vi "Create Custom Device Config Storage.vi"(8 "error in":errorcluster, 11 "Document Element":refnum<k20>) -> (0 "error out":errorcluster, 2 "Custom Device Config out":refnum<class "Custom Device Config.lvclass">, 3 "Document Element":refnum<k20>)   [LabVIEW 2024, in "Parser.lvlib" / "Custom Device Config.lvclass"]
uses:
  Custom Device Config.lvclass
  C:/dev/CD/niveristand-fpga-addon-custom-device/Source/Addon/Parser/Item/Item.lvclass
  Item/Controls/Item Type.ctl
  Property/Property.lvclass
  Custom Device Config.lvclass/Custom Device Config.ctl
  Item/Item.lvclass/Item.ctl
  Write XSDVersion.vi
  Write Version.vi
  Item/Write Child Items.vi
  Item/Write Properties.vi
  Write Name.vi
  <vilib>/xml/Close Reference(Node).vi
  <resource>/objmgr/DOMUserDefRef.rc
  <vilib>/xml/NI_XML.lvlib
  Item/Item.lvclass
  Parser.lvlib
  Channel/Channel.lvclass
  Section/Section.lvclass
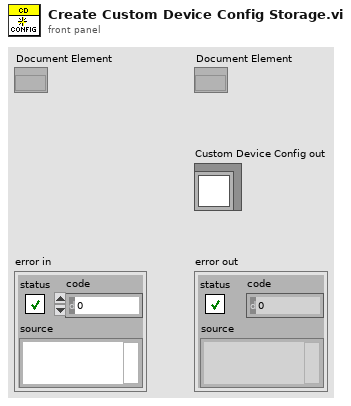
[diagram p1: front panel]
types:
  T1 = cluster{"Major":u32, " Minor":u32, " Fix":u32, "Build":u32}
  T2 = typedef "Parser.lvlib/Item.lvclass/Item Type.ctl" = enum16{"Channel", "Section"}
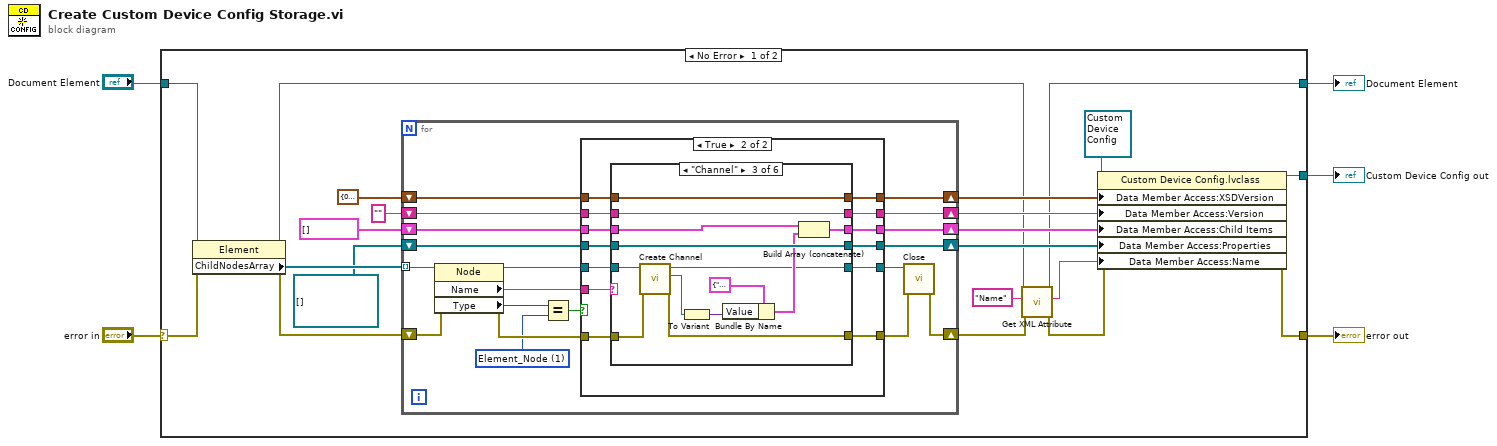
[diagram p0: block diagram]
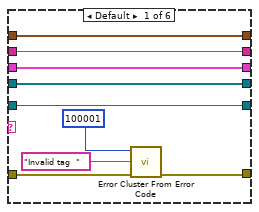
[diagram p3: hidden frame]
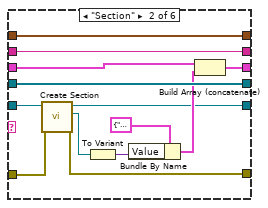
[diagram p4: hidden frame]
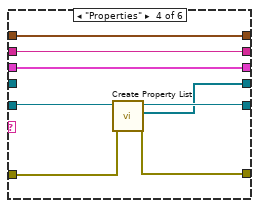
[diagram p5: hidden frame]
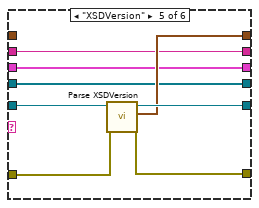
[diagram p6: hidden frame]
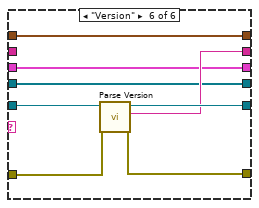
[diagram p7: hidden frame]
diagram:
  n1 = case shown="No Error" "error in" {
    selector: "error in" -> [w25 w125]
    tunnel: [w20 _] -> w3
    tunnel: [w26 w125] -> w5
    tunnel: "Document Element" -> [w19 w124]
    tunnel: [w7 w124] -> w1
    frame No Error {
      n2 = property class="Element"(reference=w19, error in=w25) -> (reference out=w8:refnum<k20>, error out=w24:errorcluster, "ChildNodesArray"=w12:refnum<k20>[])
      n3 = for {
        tunnel: w12 -> [w41] mode=indexing
        shift-right: [w44] -> w23
        shift-left: w24 -> [w45]
        shift-right: [w36] -> w18
        shift-left: T1 {"Major"=0, " Minor"=0, " Fix"=0, "Build"=0} ("XSDVersion") -> [w32]
        shift-right: [w35] -> w17
        shift-left: "" ("Version") -> [w33]
        shift-right: [w27] -> w16
        shift-left: cluster{"Item Type":T2, "Value":variant}[] [] ("Child Items") -> [w34]
        shift-right: [w29] -> w10
        shift-left: refnum<class "Property.lvclass">[] [] ("Properties") -> [w28]
        w38 = 1 items=["Element_Node"=1, "Attribute_Node"=2, "Text_Node"=3, "CDATASection_Node"=4, "EntityReference_Node"=5, "Entity_Node"=6, "ProcessingInstruction_Node"=7, "Comment_Node"=8, "Document_Node"=9, "DocumentType_Node"=10, "DocumentFragment_Node"=11, "Notation_Node"=12] ("Node Type")
        n4 = property class="Node"(reference=w41, error in=w45) -> (reference out=w39:refnum<k20>, error out=w43:errorcluster, "Name"=w31:string, "Type"=w30:i32)
        n5 = Equal?(x=w30, y=w38) -> (x = y?=w40:bool)
        n6 = case shown="True" w40 {
          tunnel: w31 -> [_ w62]
          tunnel: w39 -> [w50 w61]
          tunnel: [w50 w60] -> w37
          tunnel: w43 -> [w51 w64]
          tunnel: [w51 w63] -> w42
          tunnel: [w49 w59] -> w36
          tunnel: [w48 w58] -> w35
          tunnel: w34 -> [w46 w57]
          tunnel: w33 -> [w48 w56]
          tunnel: w32 -> [w49 w55]
          tunnel: [w47 w54] -> w29
          tunnel: w28 -> [w47 w53]
          tunnel: [w46 w52] -> w27
          frame False {
          }
          frame True {
            n7 = case shown="\"Channel\"" w62 {
              tunnel: w61 -> [w68 w84 w93 w103 w113 w121]
              tunnel: [w68 w74 w87 w102 w112 w120] -> w60
              tunnel: w64 -> [w73 w86 w99 w107 w115 w123]
              tunnel: [w72 w85 w98 w106 w114 w122] -> w63
              tunnel: [w71 w81 w97 w105 w111 w118] -> w59
              tunnel: [w70 w82 w96 w104 w110 w119] -> w58
              tunnel: w57 -> [w65 w83 w95 w100 w108 w116]
              tunnel: w56 -> [w70 w82 w96 w104 w110 _]
              tunnel: w55 -> [w71 w81 w97 w105 _ w118]
              tunnel: [w69 w80 w94 w101 w109 w117] -> w54
              tunnel: w53 -> [w69 w80 w94 _ w109 w117]
              tunnel: [w65 w76 w89 w100 w108 w116] -> w52
              frame Default {
                n8 = call <vilib>:"Error Cluster From Error Code.vi"("error in (no error)"=w73, "error message (\"\")"="Invalid tag  " ("error message (\"\")"), "error code (0)"=100001) -> ("error out"=w72:errorcluster)  [unwired: 6 in]
              }
              frame "Section" {
                n9 = call "Create Section.vi"("error in"=w86, "Node In"=w84) -> ("error out"=w85:errorcluster, "Section out"=w75:refnum<class "Section.lvclass">, "Node out"=w74:refnum<k20>)  [unwired: 7 in]
                n10 = To Variant(anything=w75) -> (Variant=w78:variant)
                n11 = Bundle By Name(cluster=cluster{"Item Type":T2, "Value":variant} {"Item Type"=enum."Section", "Value"=variant} ("Child Items"), "Value"=w78) -> (w77:cluster{"Item Type":T2, "Value":variant})
                n12 = Build Array (concatenate)(w83, w77) -> (w76:cluster{"Item Type":T2, "Value":variant}[])
              }
              frame "Channel" {
                n13 = call "Create Channel.vi"("error in"=w99, "Node In"=w93) -> ("error out"=w98:errorcluster, "Channel out"=w88:refnum<class "Channel.lvclass">, "Node out"=w87:refnum<k20>)  [unwired: 7 in]
                n14 = To Variant(anything=w88) -> (Variant=w91:variant)
                n15 = Bundle By Name(cluster=cluster{"Item Type":T2, "Value":variant} {"Item Type"=enum."Channel", "Value"=variant} ("Child Items"), "Value"=w91) -> (w90:cluster{"Item Type":T2, "Value":variant})
                n16 = Build Array (concatenate)(w95, w90) -> (w89:cluster{"Item Type":T2, "Value":variant}[])
              }
              frame "Properties" {
                n17 = call "Create Property List.vi"("error in"=w107, "Property Nodes In"=w103) -> ("error out"=w106:errorcluster, "Properties out"=w101:refnum<class "Property.lvclass">[], "Property Nodes out"=w102:refnum<k20>)  [unwired: 7 in]
              }
              frame "XSDVersion" {
                n18 = call "Parse XSDVersion.vi"("error in"=w115, "Node In"=w113) -> ("error out"=w114:errorcluster, "XSDVersion"=w111:T1, "Node Out"=w112:refnum<k20>)  [unwired: 7 in]
              }
              frame "Version" {
                n19 = call "Parse Version.vi"("error in"=w123, "Node In"=w121) -> ("error out"=w122:errorcluster, "Version"=w119:string, "Node Out"=w120:refnum<k20>)  [unwired: 7 in]
              }
            }
          }
        }
        n20 = call-poly <vilib>:"Close.vi"("error in (no error)"=w42, "node"=w37) -> ("error out"=w44:errorcluster)  [unwired: 7 in]
      }
      n21 = call "Get XML Attribute.vi"("error in"=w23, "Attribute Name"="Name", "XML Node"=w8) -> ("error out"=w22:errorcluster, "Attribute Value"=w6:string, "XML Node out"=w7:refnum<k20>)  [unwired: 6 in]
      n22 = property class="Custom Device Config.lvclass"(reference=refnum<class "Custom Device Config.lvclass"> refnum ("Parser.lvlib:Custom Device Config.lvclass"), error in=w22, "Data Member Access:XSDVersion"=w18, "Data Member Access:Version"=w17, "Data Member Access:Child Items"=w16, "Data Member Access:Properties"=w10, "Data Member Access:Name"=w6) -> (reference out=w20:refnum<class "Custom Device Config.lvclass">, error out=w26:errorcluster)
    }
    frame Error {
    }
  }
  "error out" <- w5
  "Custom Device Config out" <- w3
  "Document Element" <- w1
